vi "距离设定.vi"(0 "Digital输入":refnum<vi>, 1 "运动模式":enum32{"Absolute", "Relative"}(radio)=enum."Relative", 2 "Reset Counter":bool, 5 "reference 3":refnum<vi>, 7 "reference输入":refnum<vi>, 9 "索引":i32, 12 "设定距离":dbl=50000.0, 13 "设置速度":dbl=10000.0) -> (3 "私服使能":bool, 4 "私服使能关闭":bool, 6 "相对运动":bool, 8 "绝对运动":bool, 10 "改变速度成功":bool, 14 "当前位置":dbl, 15 "轴的状态:":string)   [LabVIEW 2016]
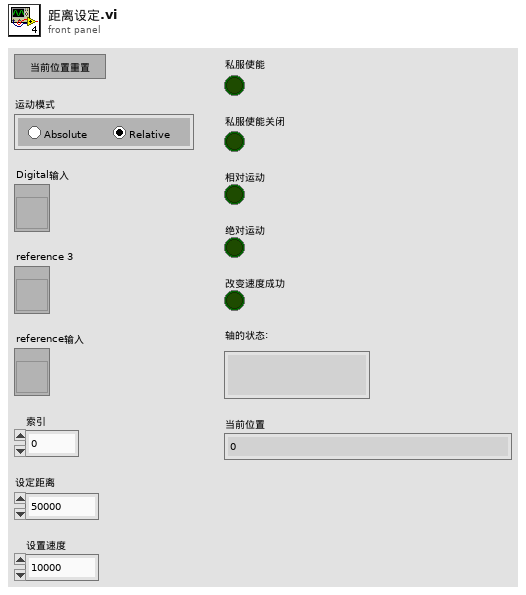
[diagram p1: front panel]
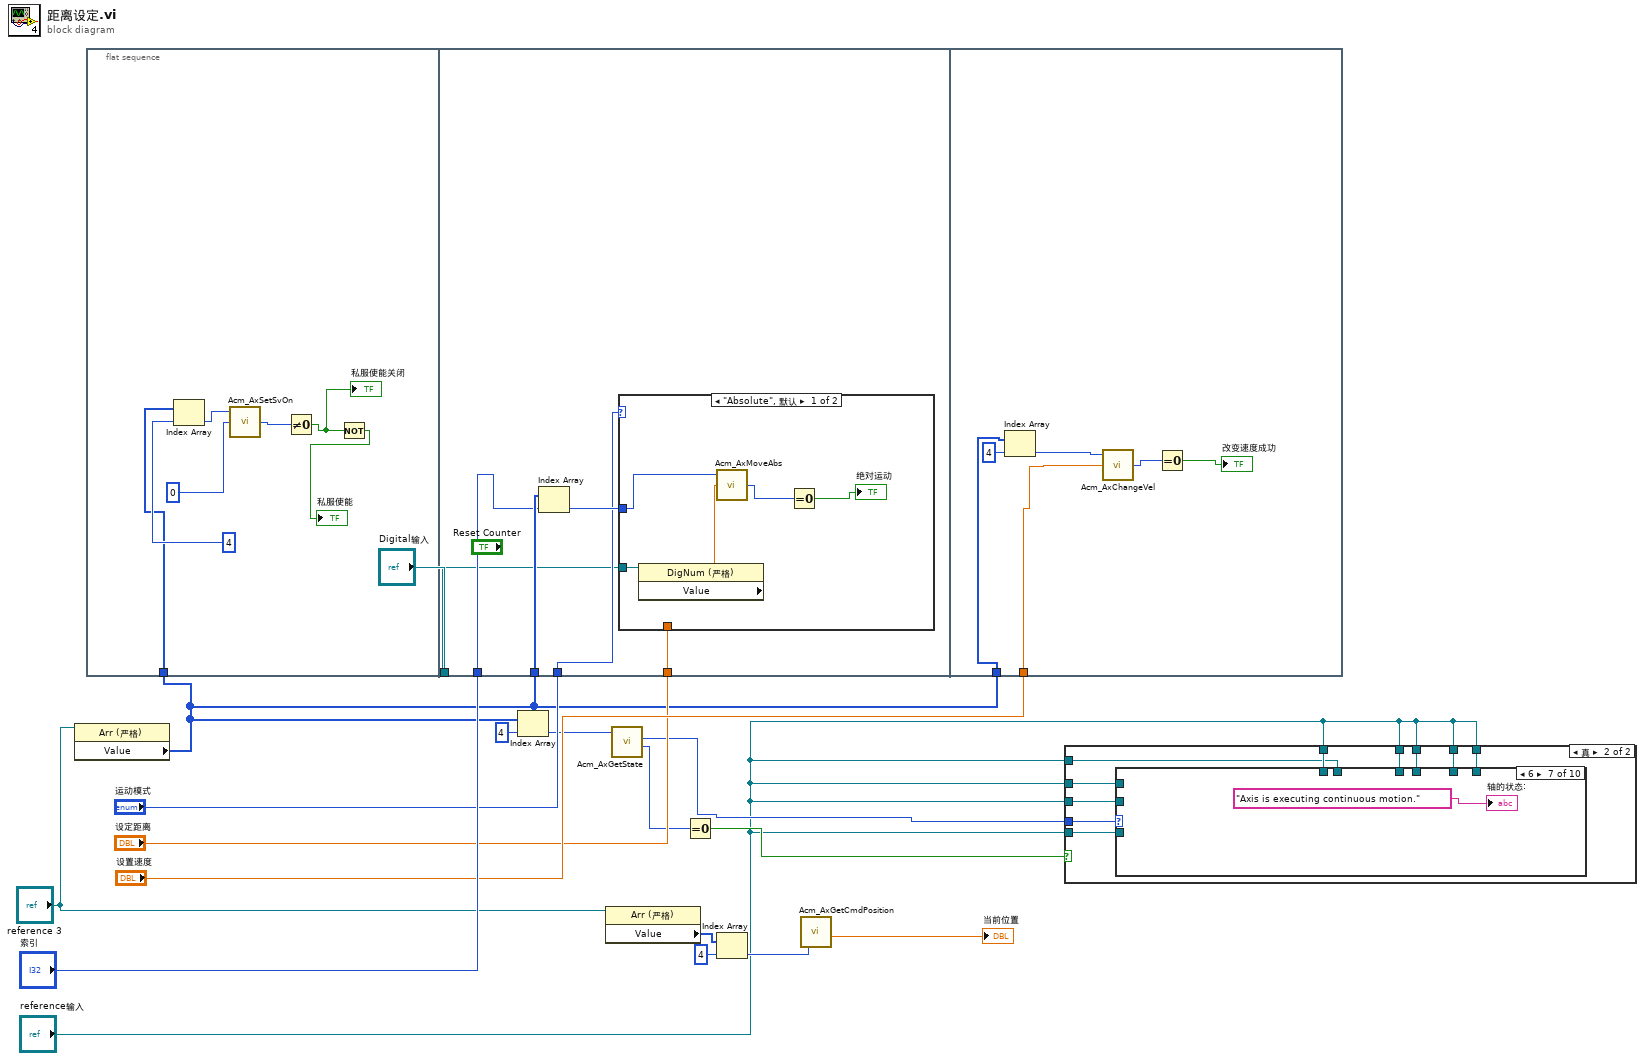
[diagram p0: block diagram]
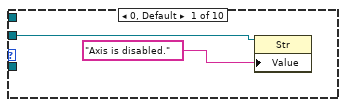
[diagram p3: hidden frame]
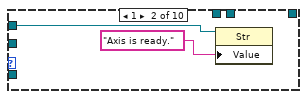
[diagram p4: hidden frame]
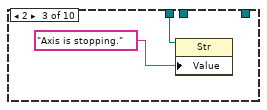
[diagram p5: hidden frame]
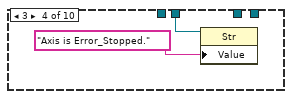
[diagram p6: hidden frame]
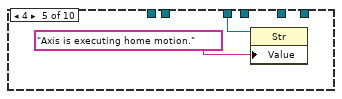
[diagram p7: hidden frame]
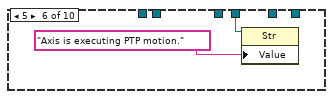
[diagram p8: hidden frame]
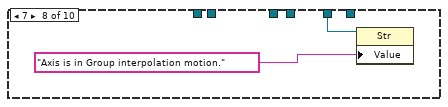
[diagram p9: hidden frame]
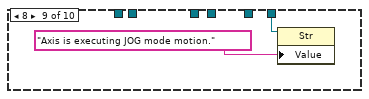
[diagram p10: hidden frame]
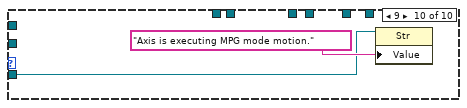
[diagram p11: hidden frame]
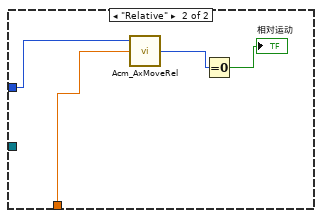
[diagram p12: hidden frame]
diagram:
  n1 = property class="Arr (严格)"(reference="reference 3") -> ("Value"=w13:u32[])  [unwired: 1 in, 2 out]
  n2 = flat-sequence {
    tunnel: w13 -> [w18]
    tunnel: w13 -> [w29]
    tunnel: "运动模式" -> [w28]
    tunnel: "设定距离" -> [w27]
    tunnel: "索引" -> [w26]
    tunnel: "Digital输入" -> [w25]
    tunnel: w13 -> [w41]
    tunnel: "设置速度" -> [w40]
    frame #0 {
      n3 = Index Array(array=w18, index=4 ("索引")) -> (element=w24:u32)
      n4 = call <userlib>:"Acm_AxSetSvOn.vi"("OnOff"=u32 0, "AxisHandle"=w24) -> ("ReturnValue"=w21:u32)  [unwired: 1 in, 2 out]
      n5 = Not Equal To 0?(x=w21) -> (x != 0?=w19:bool)
      "私服使能关闭" <- w19
      n6 = Not(x=w19) -> (.not. x?=→"私服使能":bool)
    }
    frame #1 {
      n7 = Index Array(array=w29, index=w26) -> (element=w30:u32)
      n8 = case shown="\"Absolute\", 默认" w28 {
        tunnel: w30 -> [w35 w39]
        tunnel: w27 -> [_ w36]
        tunnel: w25 -> [w31 _]
        frame "Absolute", Default {
          n9 = property class="DigNum (严格)"(reference=w31) -> ("Value"=w34:dbl)  [unwired: 1 in, 2 out]
          n10 = call <userlib>:"Acm_AxMoveAbs.vi"("Position"=w34, "AxisHandle"=w35) -> ("ReturnValue"=w33:u32)  [unwired: 1 in, 2 out]
          n11 = Equal To 0?(x=w33) -> (x = 0?=→"绝对运动":bool)
        }
        frame "Relative" {
          n12 = call <userlib>:"Acm_AxMoveRel.vi"("Distance"=w36, "AxisHandle"=w39) -> ("ReturnValue"=w38:u32)  [unwired: 1 in, 2 out]
          n13 = Equal To 0?(x=w38) -> (x = 0?=→"相对运动":bool)
        }
      }
    }
    frame #2 {
      n14 = Index Array(array=w41, index=4 ("索引")) -> (element=w44:u32)
      n15 = call <userlib>:"Acm_AxChangeVel.vi"("NewVelocity"=w40, "AxisHandle"=w44) -> ("ReturnValue"=w43:u32)  [unwired: 1 in, 2 out]
      n16 = Equal To 0?(x=w43) -> (x = 0?=→"改变速度成功":bool)
    }
  }
  n17 = Index Array(array=w13, index=4 ("索引")) -> (element=w8:u32)
  n18 = property class="Arr (严格)"(reference="reference 3") -> ("Value"=w9:u32[])  [unwired: 1 in, 2 out]
  n19 = call <userlib>:"Acm_AxGetState.vi"("AxisHandle"=w8) -> ("ReturnValue"=w6:u32, "Status"=w4:u16)  [unwired: 1 in, 2 out]
  n20 = Equal To 0?(x=w6) -> (x = 0?=w5:bool)
  n21 = Index Array(array=w9, index=4 ("索引")) -> (element=w10:u32)
  n22 = call <userlib>:"Acm_AxGetCmdPosition.vi"("AxisHandle"=w10) -> ("Position"=→"当前位置":dbl)  [unwired: 1 in, 3 out]
  n23 = case shown="真" w5 {
    tunnel: w4 -> [_ w55]
    tunnel: "reference输入" -> [_ w54]
    tunnel: "reference输入" -> [_ w53]
    tunnel: "reference输入" -> [_ w52]
    tunnel: "reference输入" -> [_ w51]
    tunnel: "reference输入" -> [_ w50]
    tunnel: "reference输入" -> [_ w49]
    tunnel: "reference输入" -> [_ w48]
    tunnel: "reference输入" -> [_ w47]
    tunnel: "reference输入" -> [_ w46]
    frame False {
    }
    frame True {
      n24 = case shown="6" w55 {
        tunnel: w54 -> [w56 _ _ _ _ _ _ _ _ _]
        tunnel: w53 -> [_ w58 _ _ _ _ _ _ _ _]
        tunnel: w52 -> [_ _ w60 _ _ _ _ _ _ _]
        tunnel: w51 -> [_ _ _ w62 _ _ _ _ _ _]
        tunnel: w50 -> [_ _ _ _ w64 _ _ _ _ _]
        tunnel: w49 -> [_ _ _ _ _ w66 _ _ _ _]
        tunnel: w48 -> [_ _ _ _ _ _ _ w69 _ _]
        tunnel: w47 -> [_ _ _ _ _ _ _ _ w71 _]
        tunnel: w46 -> [_ _ _ _ _ _ _ _ _ w73]
        frame 0, Default {
          n25 = property class="Str"(reference=w56, "Value"="Axis is disabled." ("Axis State:")) -> ()  [unwired: 1 in, 2 out]
        }
        frame 1 {
          n26 = property class="Str"(reference=w58, "Value"="Axis is ready." ("Axis State:")) -> ()  [unwired: 1 in, 2 out]
        }
        frame 2 {
          n27 = property class="Str"(reference=w60, "Value"="Axis is stopping." ("Axis State:")) -> ()  [unwired: 1 in, 2 out]
        }
        frame 3 {
          n28 = property class="Str"(reference=w62, "Value"="Axis is Error_Stopped." ("Axis State:")) -> ()  [unwired: 1 in, 2 out]
        }
        frame 4 {
          n29 = property class="Str"(reference=w64, "Value"="Axis is executing home motion." ("Axis State:")) -> ()  [unwired: 1 in, 2 out]
        }
        frame 5 {
          n30 = property class="Str"(reference=w66, "Value"="Axis is executing PTP motion." ("Axis State:")) -> ()  [unwired: 1 in, 2 out]
        }
        frame 6 {
          "轴的状态:" <- "Axis is executing continuous motion." ("Axis State:")
        }
        frame 7 {
          n31 = property class="Str"(reference=w69, "Value"="Axis is in Group interpolation motion." ("Axis State:")) -> ()  [unwired: 1 in, 2 out]
        }
        frame 8 {
          n32 = property class="Str"(reference=w71, "Value"="Axis is executing JOG mode motion." ("Axis State:")) -> ()  [unwired: 1 in, 2 out]
        }
        frame 9 {
          n33 = property class="Str"(reference=w73, "Value"="Axis is executing MPG mode motion." ("Axis State:")) -> ()  [unwired: 1 in, 2 out]
        }
      }
    }
  }
